vi "ADC to JSON.vi"(2 "dt":dbl, 4 "I_raw":waveform(dbl), 5 "Phase":dbl, 6 "U_raw":waveform(dbl), 7 "LoopId":i64, 8 "I_AC":dbl, 9 "I_DC":dbl, 10 "U_AC":dbl, 11 "U_DC":dbl) -> (0 "error out":errorcluster, 3 "JSON":string)   [LabVIEW 2014]
doc: "Building up of a complex JSON from smaller units"
uses:
  <vilib>/addons/JSON API/JSON Value/Get as JSON string.vi
  <vilib>/addons/JSON API/JSON Scalar/Set I64.vi
  <vilib>/addons/JSON API/JSON Scalar/Set DBL.vi
  <vilib>/addons/JSON API/JSON Object/Set Waveform.vi
  <vilib>/addons/JSON API/JSON Scalar/Set Timestamp.vi
  <vilib>/addons/JSON API/JSON Object/Set Object Item by name.vi
  <vilib>/addons/JSON API/JSON Value/Get Item by name array.vi
  <vilib>/addons/JSON API/JSON Value/JSON Value.lvclass
  <vilib>/addons/JSON API/Get Polymorphic/JSON GetSet.lvlib
  <vilib>/addons/JSON API/JSON Object/JSON Object.lvclass
  <vilib>/addons/JSON API/JSON Scalar/JSON Scalar.lvclass
panel:
  # "see diagram"
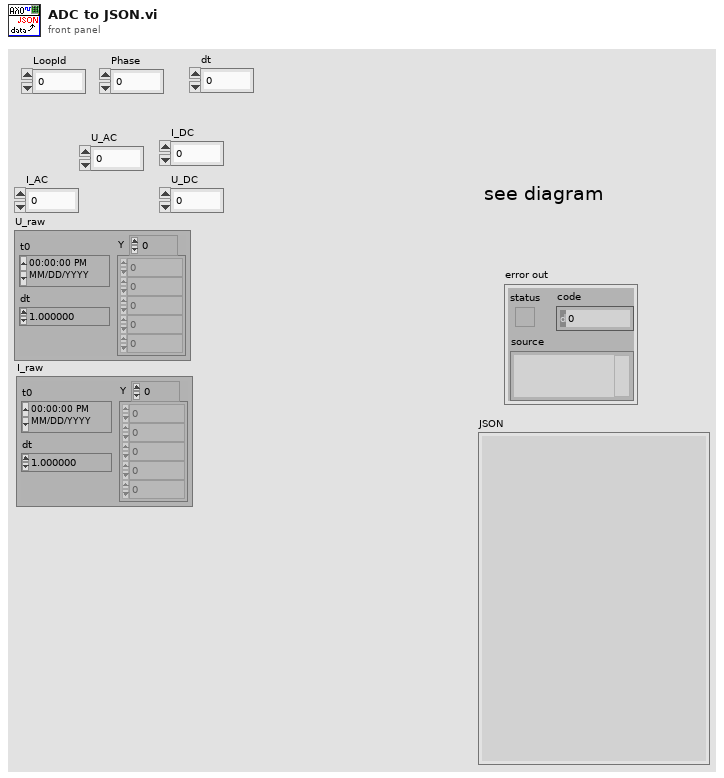
[diagram p1: front panel]
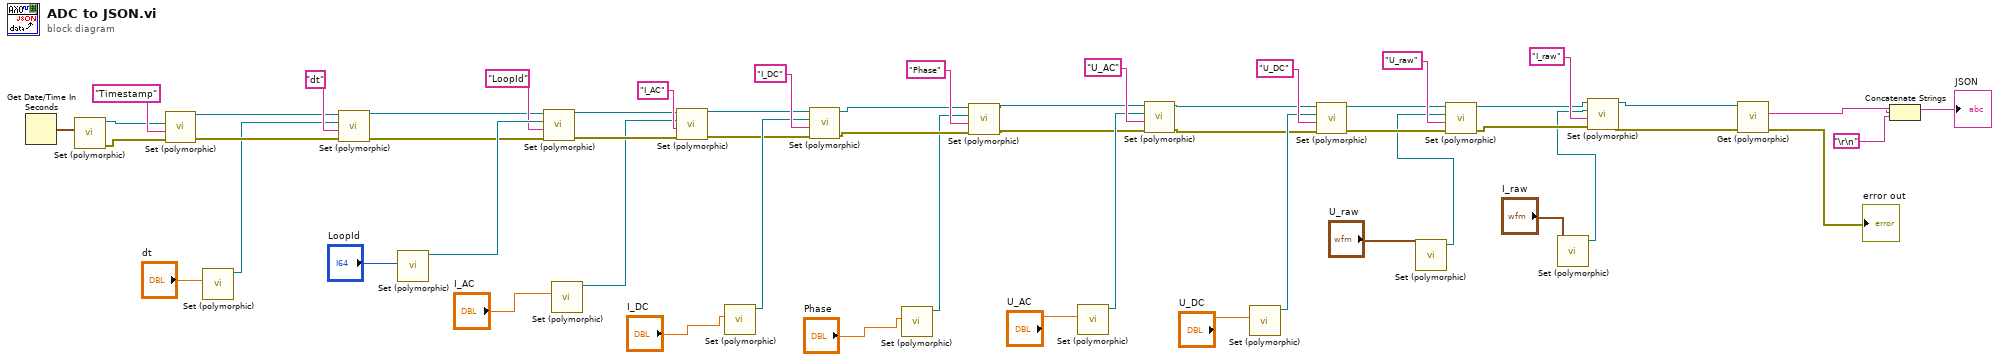
[diagram p0: block diagram]
diagram:
  n1 = Get Date/Time In Seconds() -> (seconds since 1Jan1904=w55:timestamp)
  n2 = call-poly <vilib>:"Set (polymorphic).vi"("Time Stamp"=w55) -> ("error out"=w47:errorcluster, "JSON Scalar out"=w53:refnum<class "JSON Scalar.lvclass">)  [unwired: 9 in]
  n3 = call-poly <vilib>:"Set (polymorphic).vi"("error in (no error)"=w47, "name"="Timestamp", "Value"=w53) -> ("error out"=w3:errorcluster, "JSON Object out"=w4:refnum<class "JSON Object.lvclass">)  [unwired: 6 in, 1 out]
  n4 = call-poly <vilib>:"Set (polymorphic).vi"("Numeric"="dt") -> ("JSON Scalar out"=w2:refnum<class "JSON Scalar.lvclass">)  [unwired: 9 in, 1 out]
  n5 = call-poly <vilib>:"Set (polymorphic).vi"("error in (no error)"=w3, "name"="dt", "Value"=w2, "JSON Object in"=w4) -> ("error out"=w5:errorcluster, "JSON Object out"=w6:refnum<class "JSON Object.lvclass">)  [unwired: 5 in, 1 out]
  n6 = call-poly <vilib>:"Set (polymorphic).vi"("Numeric"="LoopId") -> ("JSON Scalar out"=w50:refnum<class "JSON Scalar.lvclass">)  [unwired: 9 in, 1 out]
  n7 = call-poly <vilib>:"Set (polymorphic).vi"("error in (no error)"=w5, "name"="LoopId", "Value"=w50, "JSON Object in"=w6) -> ("error out"=w46:errorcluster, "JSON Object out"=w48:refnum<class "JSON Object.lvclass">)  [unwired: 5 in, 1 out]
  n8 = call-poly <vilib>:"Set (polymorphic).vi"("Numeric"="I_AC") -> ("JSON Scalar out"=w44:refnum<class "JSON Scalar.lvclass">)  [unwired: 9 in, 1 out]
  n9 = call-poly <vilib>:"Set (polymorphic).vi"("error in (no error)"=w46, "name"="I_AC", "Value"=w44, "JSON Object in"=w48) -> ("error out"=w39:errorcluster, "JSON Object out"=w40:refnum<class "JSON Object.lvclass">)  [unwired: 5 in, 1 out]
  n10 = call-poly <vilib>:"Set (polymorphic).vi"("Numeric"="I_DC") -> ("JSON Scalar out"=w41:refnum<class "JSON Scalar.lvclass">)  [unwired: 9 in, 1 out]
  n11 = call-poly <vilib>:"Set (polymorphic).vi"("error in (no error)"=w39, "name"="I_DC", "Value"=w41, "JSON Object in"=w40) -> ("error out"=w36:errorcluster, "JSON Object out"=w37:refnum<class "JSON Object.lvclass">)  [unwired: 5 in, 1 out]
  n12 = call-poly <vilib>:"Set (polymorphic).vi"("Numeric"="Phase") -> ("JSON Scalar out"=w34:refnum<class "JSON Scalar.lvclass">)  [unwired: 9 in, 1 out]
  n13 = call-poly <vilib>:"Set (polymorphic).vi"("error in (no error)"=w36, "name"="Phase", "Value"=w34, "JSON Object in"=w37) -> ("error out"=w29:errorcluster, "JSON Object out"=w30:refnum<class "JSON Object.lvclass">)  [unwired: 5 in, 1 out]
  n14 = call-poly <vilib>:"Set (polymorphic).vi"("Numeric"="U_AC") -> ("JSON Scalar out"=w32:refnum<class "JSON Scalar.lvclass">)  [unwired: 9 in, 1 out]
  n15 = call-poly <vilib>:"Set (polymorphic).vi"("error in (no error)"=w29, "name"="U_AC", "Value"=w32, "JSON Object in"=w30) -> ("error out"=w24:errorcluster, "JSON Object out"=w25:refnum<class "JSON Object.lvclass">)  [unwired: 5 in, 1 out]
  n16 = call-poly <vilib>:"Set (polymorphic).vi"("Numeric"="U_DC") -> ("JSON Scalar out"=w27:refnum<class "JSON Scalar.lvclass">)  [unwired: 9 in, 1 out]
  n17 = call-poly <vilib>:"Set (polymorphic).vi"("error in (no error)"=w24, "name"="U_DC", "Value"=w27, "JSON Object in"=w25) -> ("error out"=w22:errorcluster, "JSON Object out"=w21:refnum<class "JSON Object.lvclass">)  [unwired: 5 in, 1 out]
  n18 = call-poly <vilib>:"Set (polymorphic).vi"("waveform"="U_raw") -> ("JSON Object out"=w20:refnum<class "JSON Object.lvclass">)  [unwired: 9 in, 1 out]
  n19 = call-poly <vilib>:"Set (polymorphic).vi"("error in (no error)"=w22, "name"="U_raw", "Value"=w20, "JSON Object in"=w21) -> ("error out"=w17:errorcluster, "JSON Object out"=w16:refnum<class "JSON Object.lvclass">)  [unwired: 5 in, 1 out]
  n20 = call-poly <vilib>:"Set (polymorphic).vi"("waveform"="I_raw") -> ("JSON Object out"=w15:refnum<class "JSON Object.lvclass">)  [unwired: 9 in, 1 out]
  n21 = call-poly <vilib>:"Set (polymorphic).vi"("error in (no error)"=w17, "name"="I_raw", "Value"=w15, "JSON Object in"=w16) -> ("error out"=w12:errorcluster, "JSON Object out"=w13:refnum<class "JSON Object.lvclass">)  [unwired: 5 in, 1 out]
  n22 = call-poly <vilib>:"Get (polymorphic).vi"("error in (no error)"=w12, "JSON Value in"=w13) -> ("error out"=→"error out":errorcluster, "String"=w10:string)  [unwired: 8 in]
  n23 = Concatenate Strings(w10, "\r\n") -> (→"JSON":string)
